vi "Read Debug Data Event.vi"(8 "error in (no error)":errorcluster, 11 "Debug Data Event in":refnum<class "Debug Data Event.lvclass">) -> (0 "error out":errorcluster, 2 "Debug Data Event":refnum<user-event>, 3 "Debug Data Event out":refnum<class "Debug Data Event.lvclass">)   [LabVIEW 2020, in "Debug Data Event.lvclass"]
uses:
  Debug Data Event.lvclass
  Debug Message Receiver/Public/Debug Data Cluster.ctl
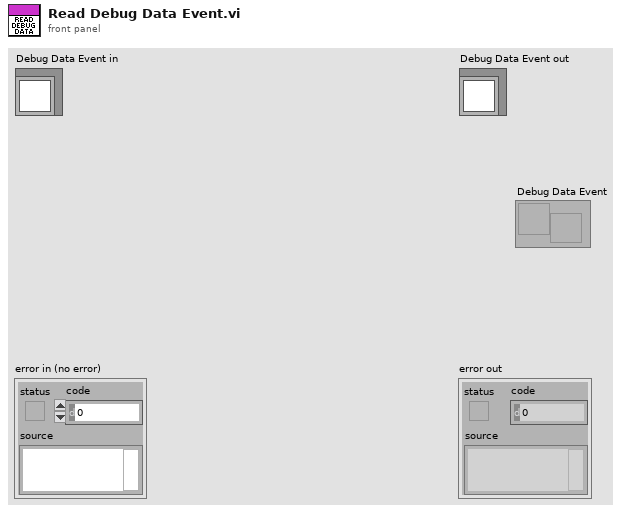
[diagram p1: front panel]
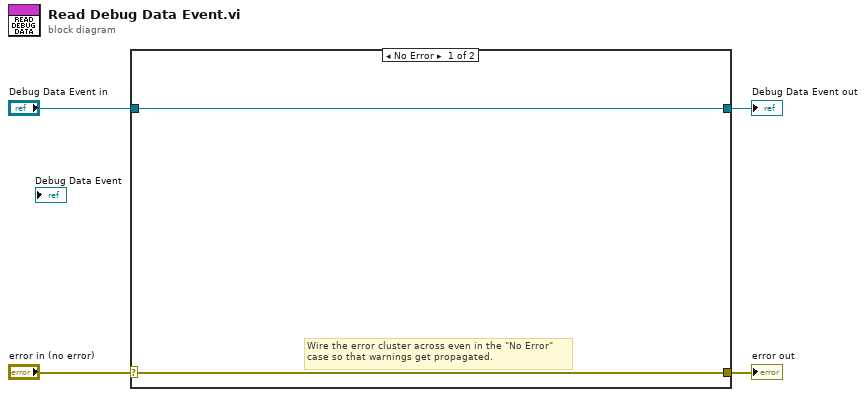
[diagram p0: block diagram]
diagram:
  n1 = case shown="No Error" "error in (no error)" {
    selector: "error in (no error)" -> [w5 w8]
    tunnel: [w5 w8] -> w3
    tunnel: [w6 w7] -> w1
    tunnel: "Debug Data Event in" -> [w6 w7]
    frame No Error {
      # "Wire the error cluster across even in the \"No Error\"\ncase so that warnings get propagated."
    }
    frame Error {
    }
  }
  "error out" <- w3
  "Debug Data Event out" <- w1
